vi "TXD_QUEUE.vi"(8 "error in (no error)":errorcluster caption="에러 입력(에러 없음)", 10 "송신문자":string, 11 "전송?":bool=TRUE) -> (0 "error out":errorcluster caption="에러 출력", 3 "queue out":refnum<queue>)   [LabVIEW 2014]
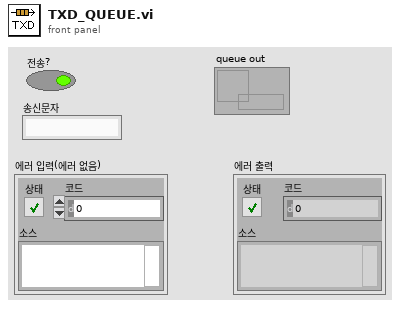
[diagram p1: front panel]
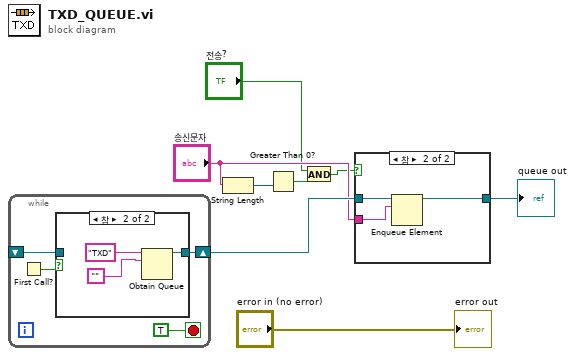
[diagram p0: block diagram]
diagram:
  n1 = while {
    shift-right: [w12] -> w8
    shift-left: _ -> [w10]
    stop <- TRUE stop-if-true
    n2 = First Call?() -> (First Call?: T/F=w9:bool)
    n3 = case shown="참" w9 {
      tunnel: [w13 w16] -> w12
      tunnel: w10 -> [w13 _]
      frame False {
      }
      frame True {
        n4 = Obtain Queue(name (unnamed)="TXD", element data type="") -> (queue out=w16:refnum<queue>)  [unwired: 3 in, 2 out]
      }
    }
  }
  n5 = String Length(string="송신문자") -> (length=w4:i32)
  n6 = Greater Than 0?(x=w4) -> (x > 0?=w3:bool)
  n7 = And(x="전송?", y=w3) -> (x .and. y?=w1:bool)
  n8 = case shown="참" w1 {
    tunnel: w8 -> [w17 w20]
    tunnel: "송신문자" -> [_ w19]
    tunnel: [w17 w18] -> w6
    frame False {
    }
    frame True {
      n9 = Enqueue Element(queue=w20, element=w19) -> (queue out=w18:refnum<queue>)  [unwired: 2 in, 2 out]
    }
  }
  "queue out" <- w6
  "error out" <- "error in (no error)"
